vi "Update Package Version from Build Rev.vi"(8 "error in":cluster{"status":bool, "code":i32, string}, 10 "Package Spec File":path, 11 "Build File":path) -> (0 "error out":errorcluster)   [LabVIEW 2011]
uses:
  <vilib>/Utility/config.llb/Read Key (Path).vi
  <userlib>/_OpenG.lib/file/file.llb/Append Path to Root if Relative - Scalar__ogtk.vi
  <vilib>/Utility/config.llb/Read Key (String).vi
  <vilib>/Utility/config.llb/Write Key (String).vi
  <vilib>/Utility/config.llb/NI_LVConfig.lvlib
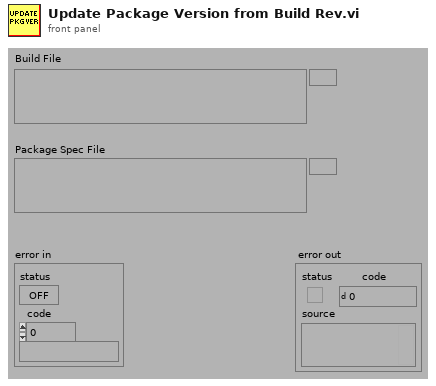
[diagram p1: front panel]
types:
  T1 = typedef "NI_LVConfig.lvlib/Config Data RefNum.ctl" = refnum<k1>
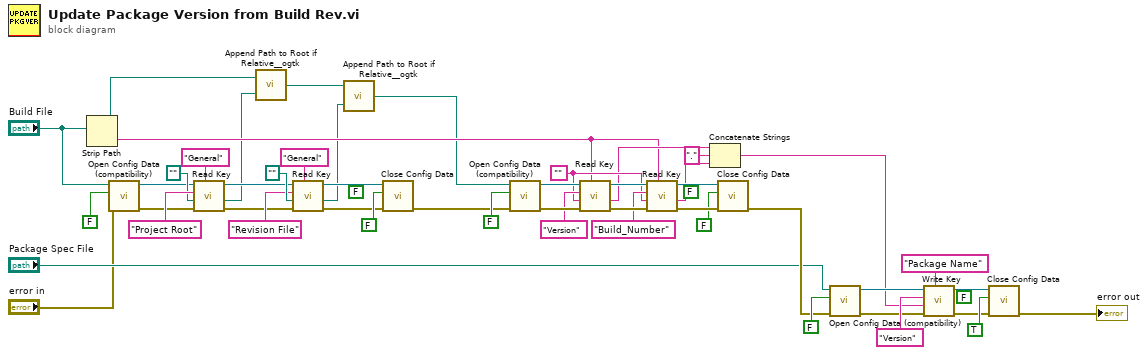
[diagram p0: block diagram]
diagram:
  (unwired) FALSE ("write configuration file? (T)")
  (unwired) FALSE ("write configuration file? (T)")
  (unwired) FALSE ("write configuration file? (T)")
  w31 = ""
  n1 = Strip Path(path="Build File") -> (stripped path=w5:path, name=w23:string)
  n2 = call <vilib>:"Open Config Data (compatibility).vi"("error in (no error)"="error in", "create file if necessary (T)"=FALSE ("create file if necessary? (T)"), "configuration file path"="Build File") -> ("error out"=w9:errorcluster, "refnum"=w6:T1)  [unwired: 6 in, 1 out]
  n3 = call-poly <vilib>:"Read Key.vi"("section"="General", "error in (no error)"=w9, "default value"=path "", "key"="Project Root", "refnum"=w6) -> ("error out"=w8:errorcluster, "value"=w4:path, "refnum out"=w7:T1)  [unwired: 3 in, 1 out]
  n4 = call-poly <userlib>:"Append Path to Root if Relative__ogtk.vi"("Absolute or Relative Path"=w4, "Root Path"=w5) -> ("Absolute or Appended Path"=w3:path)
  n5 = call-poly <vilib>:"Read Key.vi"("section"="General", "error in (no error)"=w8, "default value"=path "", "key"="Revision File", "refnum"=w7) -> ("error out"=w18:errorcluster, "value"=w2:path, "refnum out"=w17:T1)  [unwired: 3 in, 1 out]
  n6 = call-poly <userlib>:"Append Path to Root if Relative__ogtk.vi"("Absolute or Relative Path"=w2, "Root Path"=w3) -> ("Absolute or Appended Path"=w1:path)
  n7 = call <vilib>:"Close Config Data.vi"("error in (no error)"=w18, "write file if changed (T)"=FALSE ("write configuration file? (F)"), "refnum"=w17) -> ("error out"=w14:errorcluster)  [unwired: 7 in, 1 out]
  n8 = call <vilib>:"Open Config Data (compatibility).vi"("error in (no error)"=w14, "create file if necessary (T)"=FALSE ("create file if necessary? (T)"), "configuration file path"=w1) -> ("error out"=w47:errorcluster, "refnum"=w48:T1)  [unwired: 6 in, 1 out]
  n9 = call-poly <vilib>:"Read Key.vi"("section"=w23, "error in (no error)"=w47, "default value"=w31, "key"="Version", "refnum"=w48) -> ("error out"=w44:errorcluster, "value"=w30:string, "refnum out"=w45:T1)  [unwired: 3 in, 1 out]
  n10 = call-poly <vilib>:"Read Key.vi"("section"=w23, "error in (no error)"=w44, "default value"=w31, "key"="Build_Number", "refnum"=w45) -> ("error out"=w41:errorcluster, "value"=w29:string, "refnum out"=w42:T1)  [unwired: 3 in, 1 out]
  n11 = Concatenate Strings(w30, "." ("string"), w29) -> (w26:string)
  n12 = call <vilib>:"Close Config Data.vi"("error in (no error)"=w41, "write file if changed (T)"=FALSE ("write configuration file? (F)"), "refnum"=w42) -> ("error out"=w25:errorcluster)  [unwired: 7 in, 1 out]
  n13 = call <vilib>:"Open Config Data (compatibility).vi"("error in (no error)"=w25, "create file if necessary (T)"=FALSE ("create file if necessary? (T)"), "configuration file path"="Package Spec File") -> ("error out"=w33:errorcluster, "refnum"=w32:T1)  [unwired: 6 in, 1 out]
  n14 = call-poly <vilib>:"Write Key.vi"("section"="Package Name", "error in (no error)"=w33, "value"=w26, "key"="Version", "refnum"=w32) -> ("error out"=w27:errorcluster, "refnum out"=w35:T1)  [unwired: 4 in, 1 out]
  n15 = call <vilib>:"Close Config Data.vi"("error in (no error)"=w27, "write file if changed (T)"=TRUE ("write configuration file? (F)"), "refnum"=w35) -> ("error out"=→"error out":errorcluster)  [unwired: 7 in, 1 out]
